vi "Uint16Array Create (Dimensions).vi"(8 "error in (no error)":errorcluster, 10 "Array dimensions":i32[](array[numeric]), 11 "U16 array in":u16[](array[numeric])) -> (0 "error out":errorcluster, 3 "Uint16Array DVR out":refnum<data-value>)   [LabVIEW 2015, in "MDSplus.lvlib"]
uses:
  <vilib>/MDSplus/Library/MDSplus.lvlib
  <vilib>/MDSplus/Classes/Data_Class/Array_Class/Uint16Array_Class/Uint16Array.lvclass
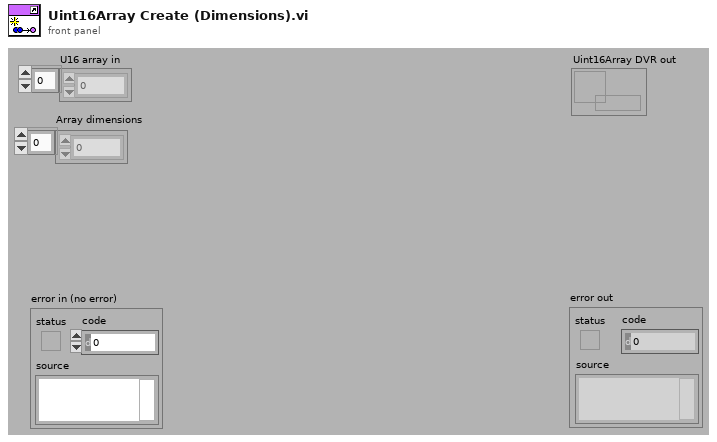
[diagram p1: front panel]
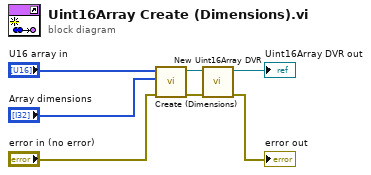
[diagram p0: block diagram]
diagram:
  n1 = call <vilib>:"Create (Dimensions).vi"("error in (no error)"="error in (no error)", "Dimensions"="Array dimensions", "U16 array in"="U16 array in") -> ("error out"=w4:errorcluster, "Uint16Array out"=w5:refnum<class "Uint16Array.lvclass">)  [unwired: 7 in]
  n2 = call <vilib>:"New Uint16Array DVR.vi"("error in (no error)"=w4, "Uint16Array in"=w5) -> ("error out"=→"error out":errorcluster, "Uint16Array DVR out"=→"Uint16Array DVR out":refnum<data-value>)  [unwired: 8 in]
